vi "Calculate Number of Remaining Samples.vi"(8 "error in (no error)":errorcluster, 11 "SV Signal in":refnum<class "SV Signal.lvclass">) -> (0 "error out":errorcluster, 3 "remaining samples":i32)   [LabVIEW 2017, in "SV Signal.lvclass"]
uses:
  <vilib>/addons/_NISVFA/_Generation/Signal Generation/SV Signal/SV Signal.lvclass
  <vilib>/addons/_NISVFA/_Generation/Signal Generation/SV Signal/SV Signal.lvclass/SV Signal.ctl
  <vilib>/addons/_NISVFA/_Generation/Signal Generation/SV Signal/sv_Generation State.ctl
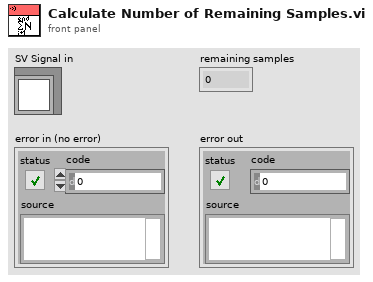
[diagram p1: front panel]
types:
  T1 = typedef "SV Signal.lvclass/sv_Generation State.ctl" = enum16{"Idle", "Ramp Up", "Pre-Measurement Settling", "Measurement", "Post-Measurement Settling", "Discrete Sweep Transition", "Ramp Down", "Update"}
  T2 = typedef "SV Signal.lvclass/sv_System Timing Model.ctl" = i64
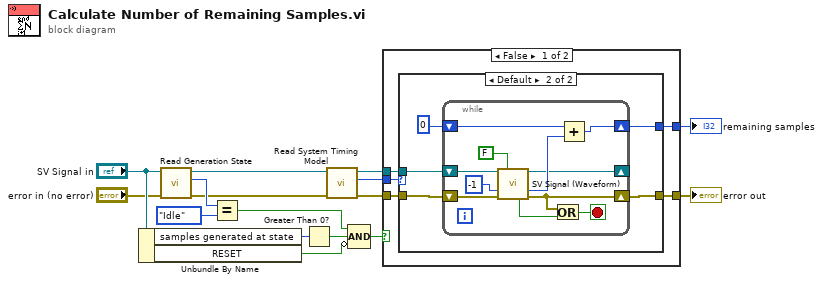
[diagram p0: block diagram]
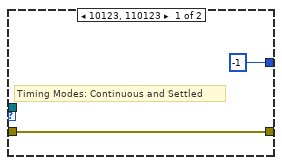
[diagram p2: hidden frame]
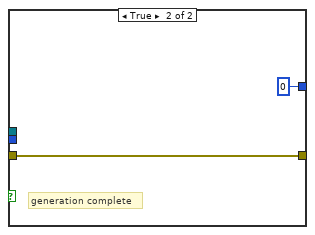
[diagram p3: hidden frame]
diagram:
  n1 = Unbundle By Name("SV Signal in") -> ("samples generated at state"=w2:u64, "RESET"=w14:bool)
  n2 = call <vilib>:"Read Generation State.vi"("error in (no error)"="error in (no error)", "SV Signal in"="SV Signal in") -> ("error out"=w5:errorcluster, "generation state"=w8:T1, "SV Signal out"=w7:refnum<class "SV Signal.lvclass">)  [unwired: 7 in]
  n3 = Equal?(x=w8, y=sv_Generation_State."Idle" ("Generation State")) -> (x = y?=w12:bool)
  n4 = Greater Than 0?(x=w2) -> (x > 0?=w1:bool)
  n5 = call <vilib>:"Read System Timing Model.vi"("error in (no error)"=w5, "signal configuration"=w7) -> ("error out"=w4:errorcluster, "system timing model"=w3:T2, "signal configuration"=w6:refnum<class "SV Signal.lvclass">)  [unwired: 7 in]
  n6 = Compound Arithmetic op=AND(w12, w1, invert w14) -> (w11:bool)
  n7 = case shown="False" w11 {
    tunnel: [w21 0 ("samples")] -> w16
    tunnel: [w20 w40] -> w15
    tunnel: w4 -> [w19 w40]
    tunnel: w6 -> [w18 _]
    tunnel: w3 -> [w17 _]
    frame False {
      n8 = case shown="Default" w17 {
        tunnel: w19 -> [w22 w28]
        tunnel: [w22 w27] -> w20
        tunnel: [-1 ("samples") w25] -> w21
        tunnel: w18 -> [_ w24]
        frame 10123, 110123 {
          # "Timing Modes: Continuous and Settled"
        }
        frame Default {
          n9 = while {
            shift-right: [w31] -> _
            shift-left: w24 -> [w33]
            shift-right: [w30] -> w27
            shift-left: w28 -> [w38]
            shift-right: [w35] -> w25
            shift-left: 0 ("samples") -> [w36]
            stop <- w37 stop-if-true
            n10 = call-dynamic "SV Signal (Waveform).vi"("signal configuration"=w33, "reset"=FALSE, "samples"=-1, "error in (no error)"=w38) -> ("signal configuration"=w31:refnum<class "SV Signal.lvclass">, "samples"=w32:i32, "done"=w29:bool, "error out"=w30:errorcluster)  [unwired: 6 in, 2 out]
            n11 = Or(x=w30, y=w29) -> (x .or. y?=w37:bool)
            n12 = Add(x=w36, y=w32) -> (x+y=w35:i32)
          }
        }
      }
    }
    frame True {
      # "generation complete"
    }
  }
  "remaining samples" <- w16
  "error out" <- w15
